vi "NI-DAQmx9237.vi"() -> (0 "error out":errorcluster)   [LabVIEW 2020]
uses:
  PWA/PWAtasksGLOBAL.vi
  <vilib>/DAQmx/configure/timing.llb/DAQmx Timing (Sample Clock).vi
  Globals/Meas_global.vi
  <resource>/objmgr/daqmx.rc
  <vilib>/DAQmx/read.llb/DAQmx Read (Analog 2D DBL NChan NSamp).vi
  <vilib>/DAQmx/create/channels.llb/DAQmx Create Channel (AI-Bridge).vi
  Sub_vis/Upload Data.ctl
panel:
  in  "units":i32(ring)=15897 items=["Volts/Volt"=15896, "mVolts/Volt"=15897, "From Custom Scale"=10065]
  in  "BridgeConfigs":T1(array[cluster]) {"voltage excitation source" items=["Internal"=10200, "External"=10167]; "bridge configuration" items=["Full Bridge"=10182, "Half Bridge"=10187, "Quarter Bridge"=10270]}
  in  "MaxRange":dbl=0.005 format="%#_13g"
  in  "MinRange":dbl=-0.005 format="%#_13g"
  out "FsReq":dbl
  out "FsRead":dbl format="%#_11g"
  out "AuditTrail":string[](array[string])
  out "TotalSampPerChanAcquired":dbl=1024.0
  out "AvailSampPerChan":u32
  out "CurrReadPos":dbl=1024.0
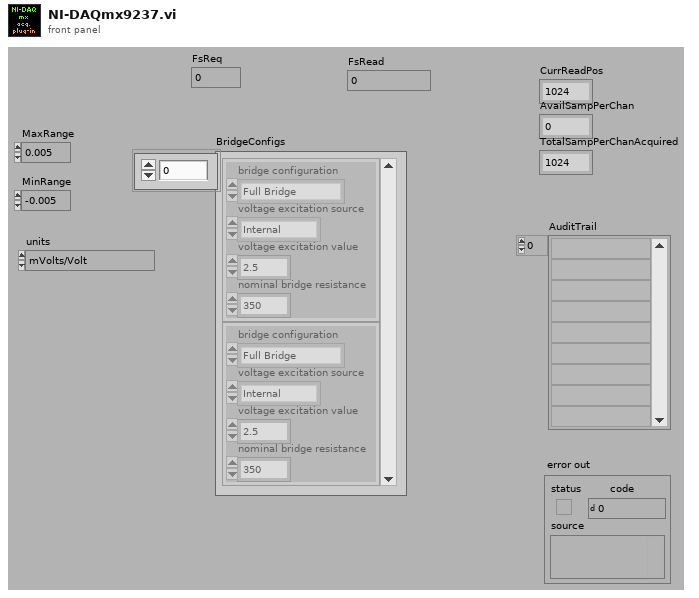
[diagram p1: front panel]
types:
  T1 = cluster{"bridge configuration":i32, "voltage excitation source":i32, "voltage excitation value":dbl, "nominal bridge resistance":dbl}[]
  T2 = typedef "Analysis_info_cluster.ctl" = cluster{"Colour":u32, "Inst type":T3, "Inst name":string, "Symbol":string, "Code name":string, "Extra Info":string, "Inst Array":T4, "Extra Titles":string[], "Extra Values":string[], "U":dbl, "u^2":dbl, "u^3":dbl, "u^4":dbl, "Skew_u":dbl, "Kurt_u":dbl, "Sd Error in Mean":dbl, "% u'/U":dbl, "X":dbl, "Y":dbl, "Z":dbl, "Timescale integral Estimate":dbl, "Sd Error in Variance":dbl, "Calib File":path, "Calib Constants":dbl[], "Output Position":bool, "Stats":enum16{"None", "Basic", "Full"}, "Av Sampling Rate":dbl, "Av No of Samples":dbl, "Total Meas Time (s)":dbl, "ADAM Ch Name":string, "Max value":dbl, "Min value":dbl, "Req Sample Rate Hz":dbl, "Sync Delay Time (s)":dbl, "Ch No":i16, "Device":string, "Use Latest Calib":bool, "Port":string, "Metadata Ch Names":string[], "Metadata Ch Values":string[], "Label":string}
  T3 = typedef "Inst_type.ctl" = enum16{"Raw voltage", "Raw with zero offsetting", "Propeller anemometer", "Pressure Transducer", "Pitot-static tube", "Hot wire", "Cross wire 1", "Cross wire 2", "Generic Linear", "Generic Polynomial", "Generic BackPoly", "Fast FID", "Thermocouple", "Cold wire", "Pulsed Wire", "LDA Vel", "LDA Tran time", "LDA Arr time", "Microphone"}
  T4 = typedef "Instrument_Array.ctl" = enum16{"PWA", "LDA", "Analogue"}
  T5 = typedef "Device ID port info.ctl" = cluster{"Ch No":i16[], "Req Sampling Rate":dbl[], "Port":string, "Index":i32[]}
  T6 = typedef "Upload Data.ctl" = enum16{"Voltage Array", "Time Trace Cluster"}
  T7 = typedef "Setup.ctl" = enum16{"Run Program", "Show Setup", "Save Current Setup", "Setup Front Panel"}
  T8 = typedef "Rendezvous RefNum" = refnum<k1>
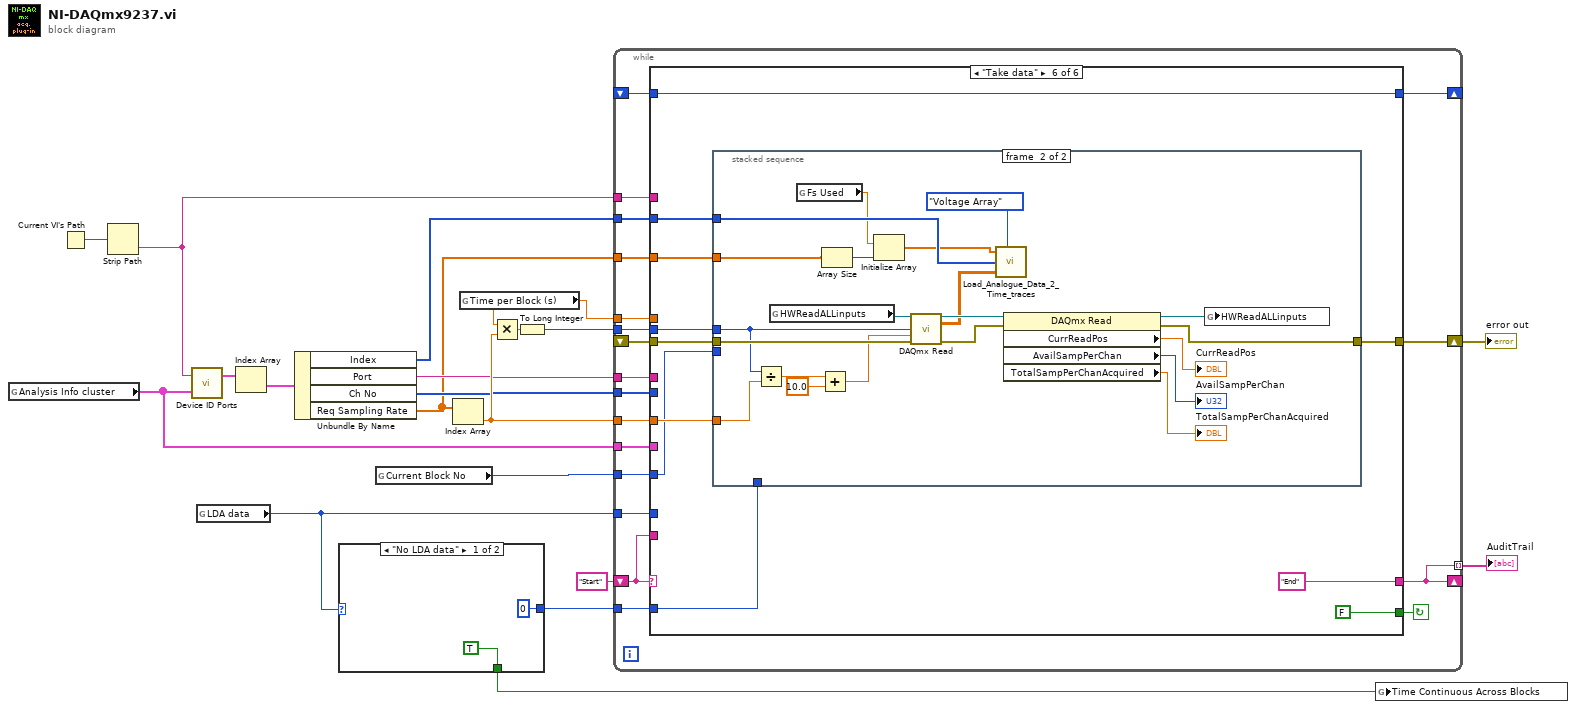
[diagram p0: block diagram]
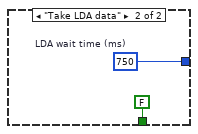
[diagram p2: hidden frame]
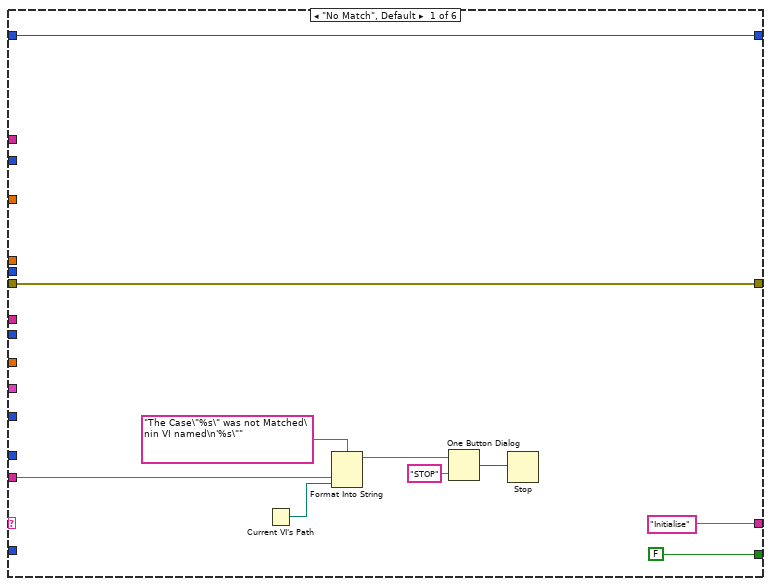
[diagram p3: hidden frame]
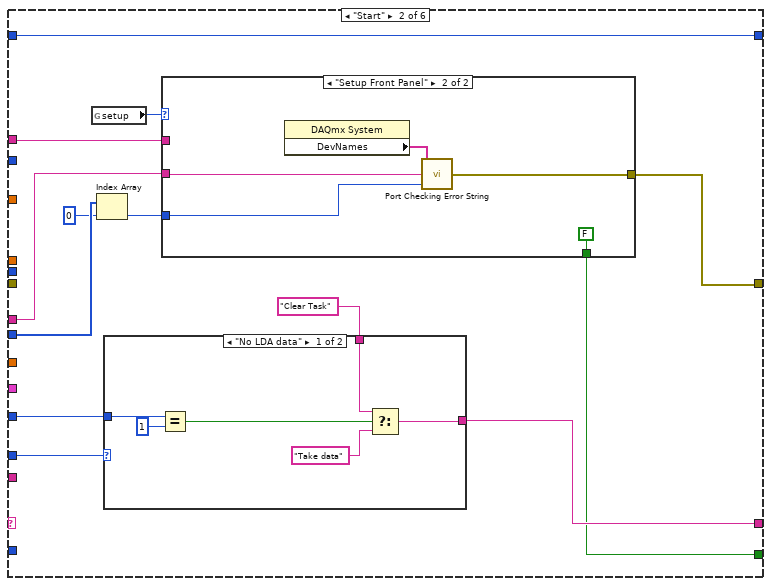
[diagram p4: hidden frame]
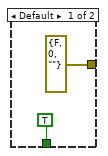
[diagram p5: hidden frame]
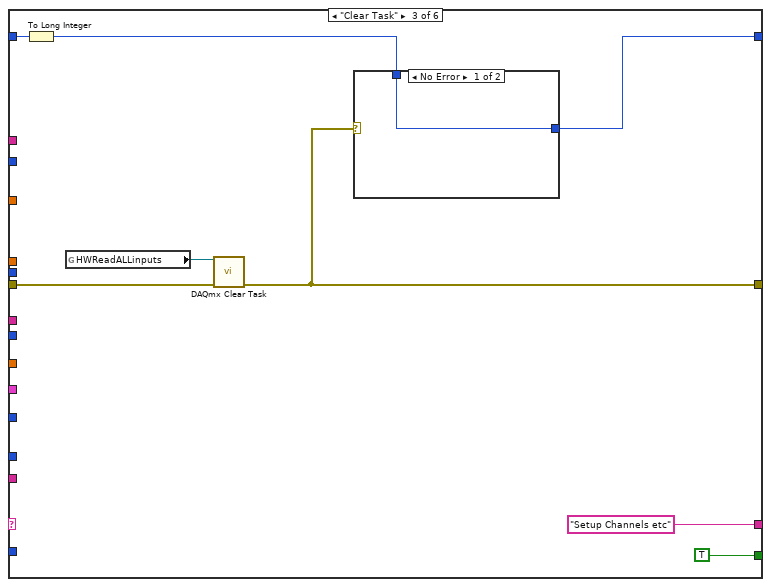
[diagram p7: hidden frame]
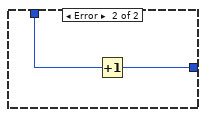
[diagram p8: hidden frame]
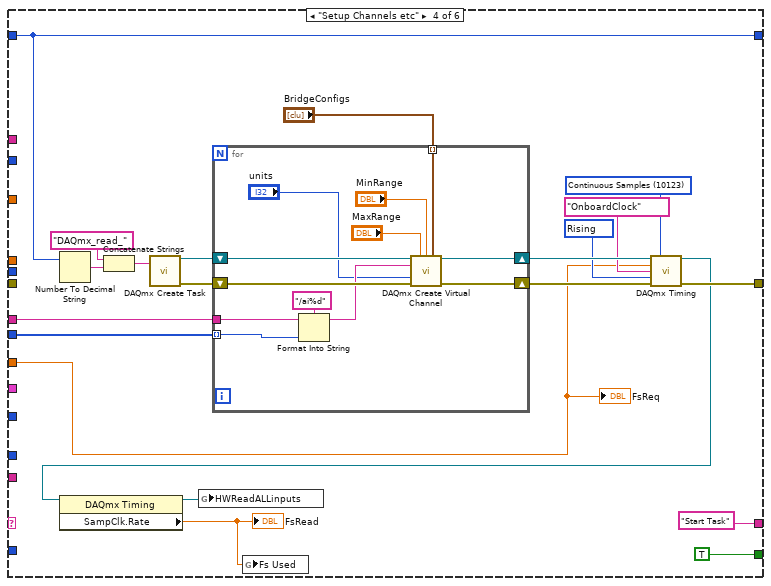
[diagram p9: hidden frame]
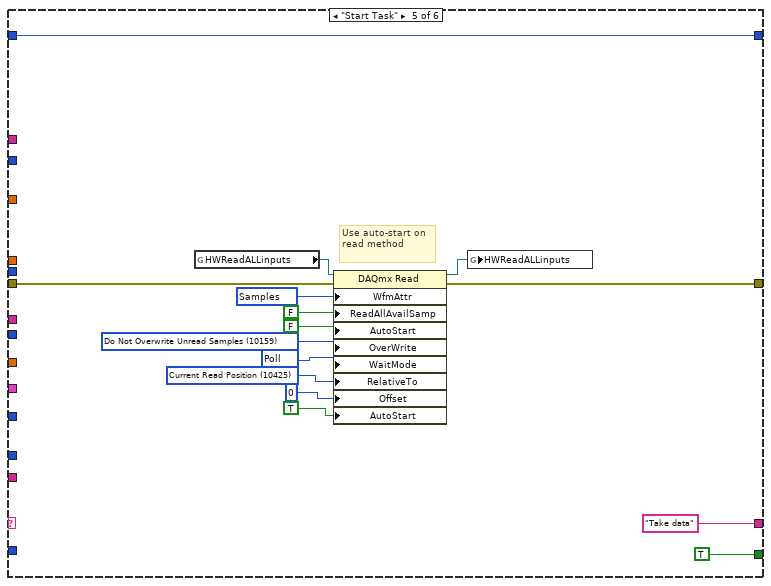
[diagram p10: hidden frame]
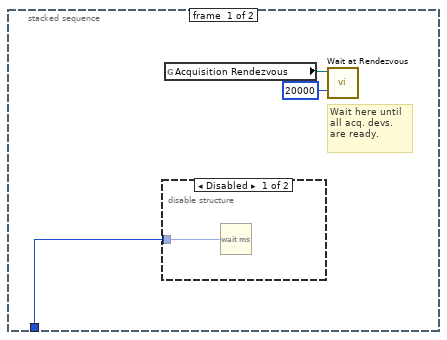
[diagram p11: hidden frame]
diagram:
  n1 = global read "Meas_global.vi" "Analysis Info cluster"() -> (w3:T2[])
  n2 = Current VI's Path() -> (path=w12:path)
  n3 = Strip Path(path=w12) -> (name=w4:string)  [unwired: 1 out]
  n4 = call "Device ID Ports.vi"("Analysis Info cluster"=w3, "Device ID"=w4) -> ("Device port info"=w10:T5[])  [unwired: 1 out]
  n5 = global read "Meas_global.vi" "LDA data"() -> (w19:enum16{"No LDA data", "Take LDA data"})
  n6 = Index Array(array=w10) -> (element=w9:T5)  [unwired: 1 in]
  n7 = Unbundle By Name(w9) -> ("Index"=w7:i32[], "Port"=w8:string, "Ch No"=w6:i16[], "Req Sampling Rate"=w5:dbl[])
  n8 = case shown="\"No LDA data\"" w19 {
    tunnel: [TRUE ("Time Continuous across Blocks") FALSE ("Time Continuous across Blocks")] -> w16
    tunnel: [u32 0 ("LDA wait time (ms)") w23] -> w15
    frame "No LDA data" {
    }
    frame "Take LDA data" {
      w23 = u32 750  # LDA wait time (ms)
    }
  }
  n9 = global read "Meas_global.vi" "Current Block No"() -> (w1:i32)
  n10 = Index Array(array=w5) -> (element=w11:dbl)  [unwired: 1 in]
  n11 = global read "Meas_global.vi" "Time per Block (s)"() -> (w2:dbl)
  n12 = Multiply(x=w2, y=w11) -> (x*y=w13:dbl)
  n13 = To Long Integer(number=w13) -> (32bit integer=w18:i32)
  n14 = while {
    shift-left: "Start" -> [w43]
    shift-right: [w34] -> _
    shift-right: [w38] -> w14
    shift-left: _ -> [w42]
    tunnel: w11 -> [w41]
    tunnel: w18 -> [w40]
    tunnel: w1 -> [w39]
    shift-right: [w37] -> _
    shift-left: _ -> [w36]
    tunnel: w19 -> [w35]
    tunnel: [w34] -> w17 mode=indexing
    tunnel: w15 -> [w33]
    tunnel: w6 -> [w32]
    tunnel: w8 -> [w31]
    tunnel: w5 -> [w30]
    tunnel: w7 -> [w29]
    tunnel: w4 -> [w28]
    tunnel: w3 -> [w27]
    tunnel: w2 -> [w25]
    stop <- w26 continue-if-true
    n15 = case shown="\"Take data\"" w43 {
      tunnel: [FALSE w54 TRUE TRUE TRUE FALSE] -> w26
      tunnel: ["Initialise" w65 "Setup Channels etc" "Start Task" "Take data" "End"] -> w34
      tunnel: w43 -> [w48 _ _ _ _ _]
      tunnel: [w45 w55 w84 w106 w126 w141] -> w38
      tunnel: w42 -> [w45 _ w85 _ w138 w150]
      tunnel: w41 -> [_ _ _ w99 _ w146]
      tunnel: w40 -> [_ _ _ _ _ w145]
      tunnel: w39 -> [_ w63 _ _ _ w140]
      tunnel: [w44 w64 w83 w98 w136 w147] -> w37
      tunnel: w36 -> [w44 w64 w82 w98 w136 w147]
      tunnel: w35 -> [_ w62 _ _ _ _]
      tunnel: w33 -> [_ _ _ _ _ w144]
      tunnel: w32 -> [_ w58 _ w96 _ _]
      tunnel: w31 -> [_ w59 _ w95 _ _]
      tunnel: w30 -> [_ _ _ _ _ w143]
      tunnel: w29 -> [_ _ _ _ _ w142]
      tunnel: w28 -> [_ w61 _ _ _ _]
      tunnel: w27 -> [_ _ _ _ _ _]
      tunnel: w25 -> [_ _ _ _ _ _]
      frame "No Match", Default {
        n16 = Current VI's Path() -> (path=w47:path)
        n17 = Format Into String(format string="The Case\"%s\" was not Matched\nin VI named\n'%s\"" ("Format String"), w48, w47) -> (resulting string=w51:string)  [unwired: 2 in, 1 out]
        n18 = One Button Dialog(message=w51, button name ("OK")="STOP") -> (true=w49:bool)
        n19 = Stop(stop? (T)=w49) -> ()
      }
      frame "Start" {
        n20 = global read "Meas_global.vi" "setup"() -> (w60:T7)
        n21 = Index Array(array=w58, index=0) -> (element=w56:i16)
        n22 = case shown="\"No LDA data\"" w62 {
          tunnel: "Clear Task" -> [w79 w80]
          tunnel: [w77 w80] -> w65
          tunnel: w63 -> [w76 _]
          frame "No LDA data" {
            n23 = Equal?(x=w76, y=1) -> (x = y?=w74:bool)
            n24 = Select(t=w79, s=w74, f="Take data") -> (s? t:f=w77:string)
          }
          frame "Take LDA data" {
          }
        }
        n25 = case shown="\"Setup Front Panel\"" w60 {
          tunnel: w61 -> [_ _]
          tunnel: w59 -> [_ w71]
          tunnel: w56 -> [_ w72]
          tunnel: [errorcluster {"status"=FALSE, "code"=0, "source"=""} ("error out") w70] -> w55
          tunnel: [TRUE FALSE] -> w54
          frame Default {
          }
          frame "Setup Front Panel" {
            n26 = property class="DAQmx System"() -> ("DevNames"=w73:tag[])  [unwired: 2 in, 2 out]
            n27 = call "Port Checking Error String.vi"("Ch Index"=w72, "Port"=w71, "Available Ports"=w73) -> ("error out"=w70:errorcluster)  [unwired: 1 in]
          }
        }
      }
      frame "Clear Task" {
        n28 = To Long Integer(number=w82) -> (32bit integer=w81:i32)
        n29 = global read "PWAtasksGLOBAL.vi" "HWReadALLinputs"() -> (w86:refnum<k21>)
        n30 = call <vilib>:"DAQmx Clear Task.vi"("task in"=w86, "error in"=w85) -> ("error out"=w84:errorcluster)  [unwired: 13 out]
        n31 = case shown="No Error" w84 {
          tunnel: [w89 w90] -> w83
          tunnel: w81 -> [w89 w91]
          frame No Error {
          }
          frame Error {
            n32 = Increment(x=w91) -> (x+1=w90:i32)
          }
        }
      }
      frame "Setup Channels etc" {
        w104 = 10280 items=["Rising"=10280, "Falling"=10171] ("active edge")
        w109 = 10123 items=["Finite Samples"=10178, "Continuous Samples"=10123, "Hardware Timed Single Point"=12522] ("sample mode")
        n33 = Number To Decimal String(number=w98) -> (decimal integer string=w97:string)  [unwired: 1 in]
        n34 = Concatenate Strings("DAQmx_read_" ("new task name"), w97) -> (w100:string)
        n35 = call <vilib>:"DAQmx Create Task.vi"("new task name"=w100) -> ("task out"=w107:refnum<k21>, "error out"=w110:errorcluster)  [unwired: 4 in, 9 out]
        n36 = for {
          shift-right: [w123] -> w108
          shift-left: w107 -> [w124]
          shift-right: [w121] -> w111
          shift-left: w110 -> [w122]
          tunnel: w96 -> [w118] mode=indexing
          tunnel: w95 -> [w117]
          tunnel: "BridgeConfigs" -> [w113] mode=indexing
          n37 = Format Into String(format string="/ai%d", initial string=w117, w118) -> (resulting string=w119:string)  [unwired: 1 in, 1 out]
          n38 = call-poly <vilib>:"DAQmx Create Virtual Channel.vi"("task in"=w124, "maximum value"="MaxRange", "minimum value"="MinRange", "bridge information"=w113, "physical channels"=w119, "units"="units", "error in"=w122) -> ("task out"=w123:refnum<k21>, "error out"=w121:errorcluster)  [unwired: 2 in, 5 out]
        }
        n39 = call-poly <vilib>:"DAQmx Timing.vi"("task/channels in"=w108, "sample mode"=w109, "rate"=w99, "source"=tag "OnboardClock", "active edge"=w104, "error in"=w111) -> ("task out"=w105:refnum<k21>, "error out"=w106:errorcluster)  [unwired: 1 in, 7 out]
        n40 = property class="DAQmx Timing"(reference=w105) -> (reference out=w94:refnum<k21>, "SampClk.Rate"=w93:dbl)  [unwired: 1 in, 1 out]
        "FsRead" <- w93
        n41 = global write "PWAtasksGLOBAL.vi" "HWReadALLinputs"(w94) -> ()
        n42 = global write "Meas_global.vi" "Fs Used"(w93) -> ()
        "FsReq" <- w99
      }
      frame "Start Task" {
        w130 = 10425 items=["First Sample"=10424, "Current Read Position"=10425, "Reference Trigger"=10426, "First Pretrigger Sample"=10427, "Most Recent Sample"=10428] ("RelativeTo")
        w131 = 12524 items=["Wait For Interrupt"=12523, "Poll"=12524, "Yield"=12525, "Sleep"=12547] ("WaitMode")
        w132 = 10159 items=["Overwrite Unread Samples"=10252, "Do Not Overwrite Unread Samples"=10159] ("OverWrite")
        w134 = 10287 items=["Samples"=10287, "Samples and Timing"=10140, "Samples, Timing, and Attributes"=10141] ("WfmAttr")
        # "Use auto-start on read method"
        n43 = global read "PWAtasksGLOBAL.vi" "HWReadALLinputs"() -> (w128:refnum<k21>)
        n44 = property class="DAQmx Read"(reference=w128, error in=w138, "WfmAttr"=w134, "ReadAllAvailSamp"=FALSE, "AutoStart"=FALSE, "OverWrite"=w132, "WaitMode"=w131, "RelativeTo"=w130, "Offset"=0, "AutoStart"=TRUE) -> (reference out=w127:refnum<k21>, error out=w126:errorcluster)
        n45 = global write "PWAtasksGLOBAL.vi" "HWReadALLinputs"(w127) -> ()
      }
      frame "Take data" {
        n46 = stacked-sequence {
          tunnel: w150 -> [_ w175]
          tunnel: w146 -> [_ w161]
          tunnel: w145 -> [_ w164]
          tunnel: [_ w163] -> w141
          tunnel: w144 -> [w153 _]
          tunnel: w143 -> [_ w159]
          tunnel: w142 -> [_ w160]
          tunnel: w140 -> [_ _]
          frame #0 {
            # "Wait here until all acq. devs. are ready."
            n47 = disable-structure shown="Disabled" {
              disable-tunnel: w153 -> [w154 _]
              frame Disabled {
                n48 = Wait (ms)(milliseconds to wait=w154) -> ()  [unwired: 1 out]
              }
              frame Enabled {
              }
            }
            n49 = global read "Meas_global.vi" "Acquisition Rendezvous"() -> (w152:T8)
            n50 = call <vilib>:"Wait at Rendezvous.vi"("ms timeout (-1)"=20000, "rendezvous"=w152) -> ()  [unwired: 3 in, 3 out]
          }
          frame #1 {
            n51 = Divide(x=w164, y=w161) -> (x/y=w167:dbl)
            n52 = global read "PWAtasksGLOBAL.vi" "HWReadALLinputs"() -> (w169:refnum<k21>)
            n53 = global read "Meas_global.vi" "Fs Used"() -> (w156:dbl)
            n54 = Add(x=w167, y=10.0) -> (x+y=w165:dbl)
            n55 = Array Size(array=w159) -> (size(s)=w158:i32)
            n56 = Initialize Array(w156, w158) -> (w157:dbl[])
            n57 = call-poly <vilib>:"DAQmx Read.vi"("task/channels in"=w169, "number of samples per channel"=w164, "timeout"=w165, "error in"=w175) -> ("task out"=w172:refnum<k21>, "data"=w162:dbl[][], "error out"=w168:errorcluster)  [unwired: 9 out]
            n58 = call "Load_Analogue_Data_2_Time_traces.vi"("Sampling Rate (Hz)"=w157, "Mode"=Upload_Data."Voltage Array", "Index"=w160, "Voltage Array"=w162) -> ()  [unwired: 3 in]
            n59 = property class="DAQmx Read"(reference=w172, error in=w168) -> (reference out=w171:refnum<k21>, error out=w163:errorcluster, "CurrReadPos"=→"CurrReadPos":dbl, "AvailSampPerChan"=→"AvailSampPerChan":u32, "TotalSampPerChanAcquired"=→"TotalSampPerChanAcquired":dbl)
            n60 = global write "PWAtasksGLOBAL.vi" "HWReadALLinputs"(w171) -> ()
          }
        }
      }
    }
  }
  "error out" <- w14
  "AuditTrail" <- w17
  n61 = global write "Meas_global.vi" "Time Continuous Across Blocks"(w16) -> ()
